vi "Abilitazione procedura torsiometro.vi"() -> (2 "Procedura abilitata":bool)   [LabVIEW 2019]
panel:
  out "Boolean":bool
  in  "OK Button":bool
  in  "Selettore":bool
  # "ABILITARE LA PROCEDURA ?"
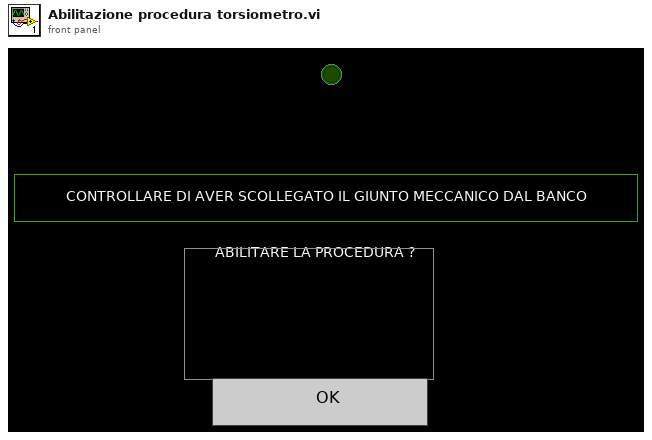
[diagram p1: front panel]
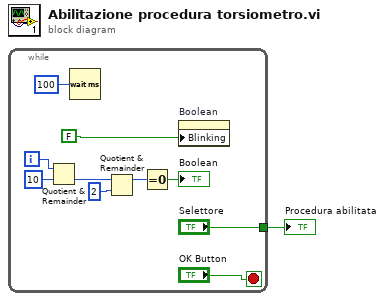
[diagram p0: block diagram]
diagram:
  n1 = while {
    tunnel: ["Selettore"] -> w1
    i -> [w7]
    stop <- "OK Button" stop-if-true
    n2 = Quotient & Remainder(x=w7, y=10) -> (floor(x/y)=w5:i32)  [unwired: 1 out]
    n3 = Wait (ms)(milliseconds to wait=u32 100) -> ()  [unwired: 1 out]
    n4 = Quotient & Remainder(x=w5, y=2) -> (x-y*floor(x/y)=w3:i32)  [unwired: 1 out]
    n5 = Equal To 0?(x=w3) -> (x = 0?=→"Boolean":bool)
    n6 = property on="Boolean" class="Bool (strict)"("Blinking"=FALSE) -> ()  [unwired: 2 in, 2 out]
  }
  "Procedura abilitata" <- w1
